vi "3DOFChairControlRebuild.vi"(9 "Scaling Factor":i32=10, 10 "Current Coord":cluster{"x (mm)":dbl, "y (mm)":dbl}={"x (mm)"=-200.0, "y (mm)"=200.0}, 11 "Previous Coord":cluster{"x (mm)":dbl, "y (mm)":dbl}) -> (0 "2D Picture 2":picture, 1 "theta3":dbl=nan, 2 "theta2":dbl=nan, 3 "theta1":dbl=nan)   [LabVIEW 2024]
uses:
  <userlib>/SerialVIs/subs/portX.xctl
panel:
  out "Coords for Sim":dbl[][](array[numeric])=[[-83.72269481496227, 7.427522229338194], [-60.199998575251854, 103.32411915468035], [-140.03201198405128, 16.093208020279867], [-16.82765846644173, 5.829527542811121], [34.47637796621948, -131.42242211582163], [68.40773502811334, 59.4509273398248], [141.31983353358055, 21.39471366409613], [101.5494686808696, 72.90895747770806], [-106.74616173728506, 110.28365634864979], [-65.90786459398325, 103.0414116639924], [-153.25841815303286, 18.106369867448336], [-11.71245505129427, 112.39652890839193], [20.969703171021592, 37.88273640369408]]
  out "output cluster":cluster{"x (mm)":dbl, "y (mm)":dbl}={"x (mm)"=-118.0, "y (mm)"=118.0}
  out "Array":dbl[](array[numeric])=[-118.0, 118.0]
  in  "Chair Back L":dbl=40.0
  out "result string 2":string="servo1.write(NaN)\nservo2.write(NaN)\nservo3.write(NaN)"
  in  "Chair Seat L":dbl=40.0
  in  "L 1":dbl=80.0
  in  "L2":dbl=80.0
  out "Interpolated Coords":dbl[][](array[numeric])=[[0.0, 0.0], [-2.0, 2.0], [-4.0, 4.0], [-6.0, 6.0], [-8.0, 8.0], [-10.0, 10.0], [-12.0, 12.0], [-14.000000000000002, 14.000000000000002], [-16.0, 16.0], [-18.0, 18.0], [-20.0, 20.0], [-22.0, 22.0], [-24.0, 24.0], [-26.0, 26.0], [-28.000000000000004, 28.000000000000004], [-30.0, 30.0], [-32.0, 32.0], [-34.0, 34.0], [-36.0, 36.0], [-38.0, 38.0], [-40.0, 40.0], [-42.0, 42.0], [-44.0, 44.0], [-46.0, 46.0], [-48.0, 48.0], [-50.0, 50.0], [-52.0, 52.0], [-54.0, 54.0], [-56.00000000000001, 56.00000000000001], [-57.99999999999999, 57.99999999999999], [-60.0, 60.0], [-62.0, 62.0], [-64.0, 64.0], [-66.0, 66.0], [-68.0, 68.0], [-70.0, 70.0], [-72.0, 72.0], [-74.0, 74.0], [-76.0, 76.0], [-78.0, 78.0], [-80.0, 80.0], [-82.0, 82.0], [-84.0, 84.0], [-86.0, 86.0], [-88.0, 88.0], [-90.0, 90.0], [-92.0, 92.0], [-94.0, 94.0], [-96.0, 96.0], [-98.0, 98.0], [-100.0, 100.0], [-102.0, 102.0], [-104.0, 104.0], [-106.0, 106.0], [-108.0, 108.0], [-110.00000000000001, 110.00000000000001], [-112.00000000000001, 112.00000000000001], [-113.99999999999999, 113.99999999999999], [-115.99999999999999, 115.99999999999999], [-118.0, 118.0], [-120.0, 120.0], [-122.0, 122.0], [-124.0, 124.0], [-126.0, 126.0], [-128.0, 128.0], [-130.0, 130.0], [-132.0, 132.0], [-134.0, 134.0], [-136.0, 136.0], [-138.0, 138.0], [-140.0, 140.0], [-142.0, 142.0], [-144.0, 144.0], [-146.0, 146.0], [-148.0, 148.0], [-150.0, 150.0], [-152.0, 152.0], [-154.0, 154.0], [-156.0, 156.0], [-158.0, 158.0], [-160.0, 160.0], [-162.0, 162.0], [-164.0, 164.0], [-166.0, 166.0], [-168.0, 168.0], [-170.0, 170.0], [-172.0, 172.0], [-174.0, 174.0], [-176.0, 176.0], [-178.0, 178.0], [-180.0, 180.0], [-182.0, 182.0], [-184.0, 184.0], [-186.0, 186.0], [-188.0, 188.0], [-190.0, 190.0], [-192.0, 192.0], [-194.0, 194.0], [-196.0, 196.0], [-198.0, 198.0], [-200.0, 200.0]]
  in  "portX":refnum<visa-resource-name>(xcontrol)="ASRL4"
  out "reply":string="\r\n>>> \r\n>>> "
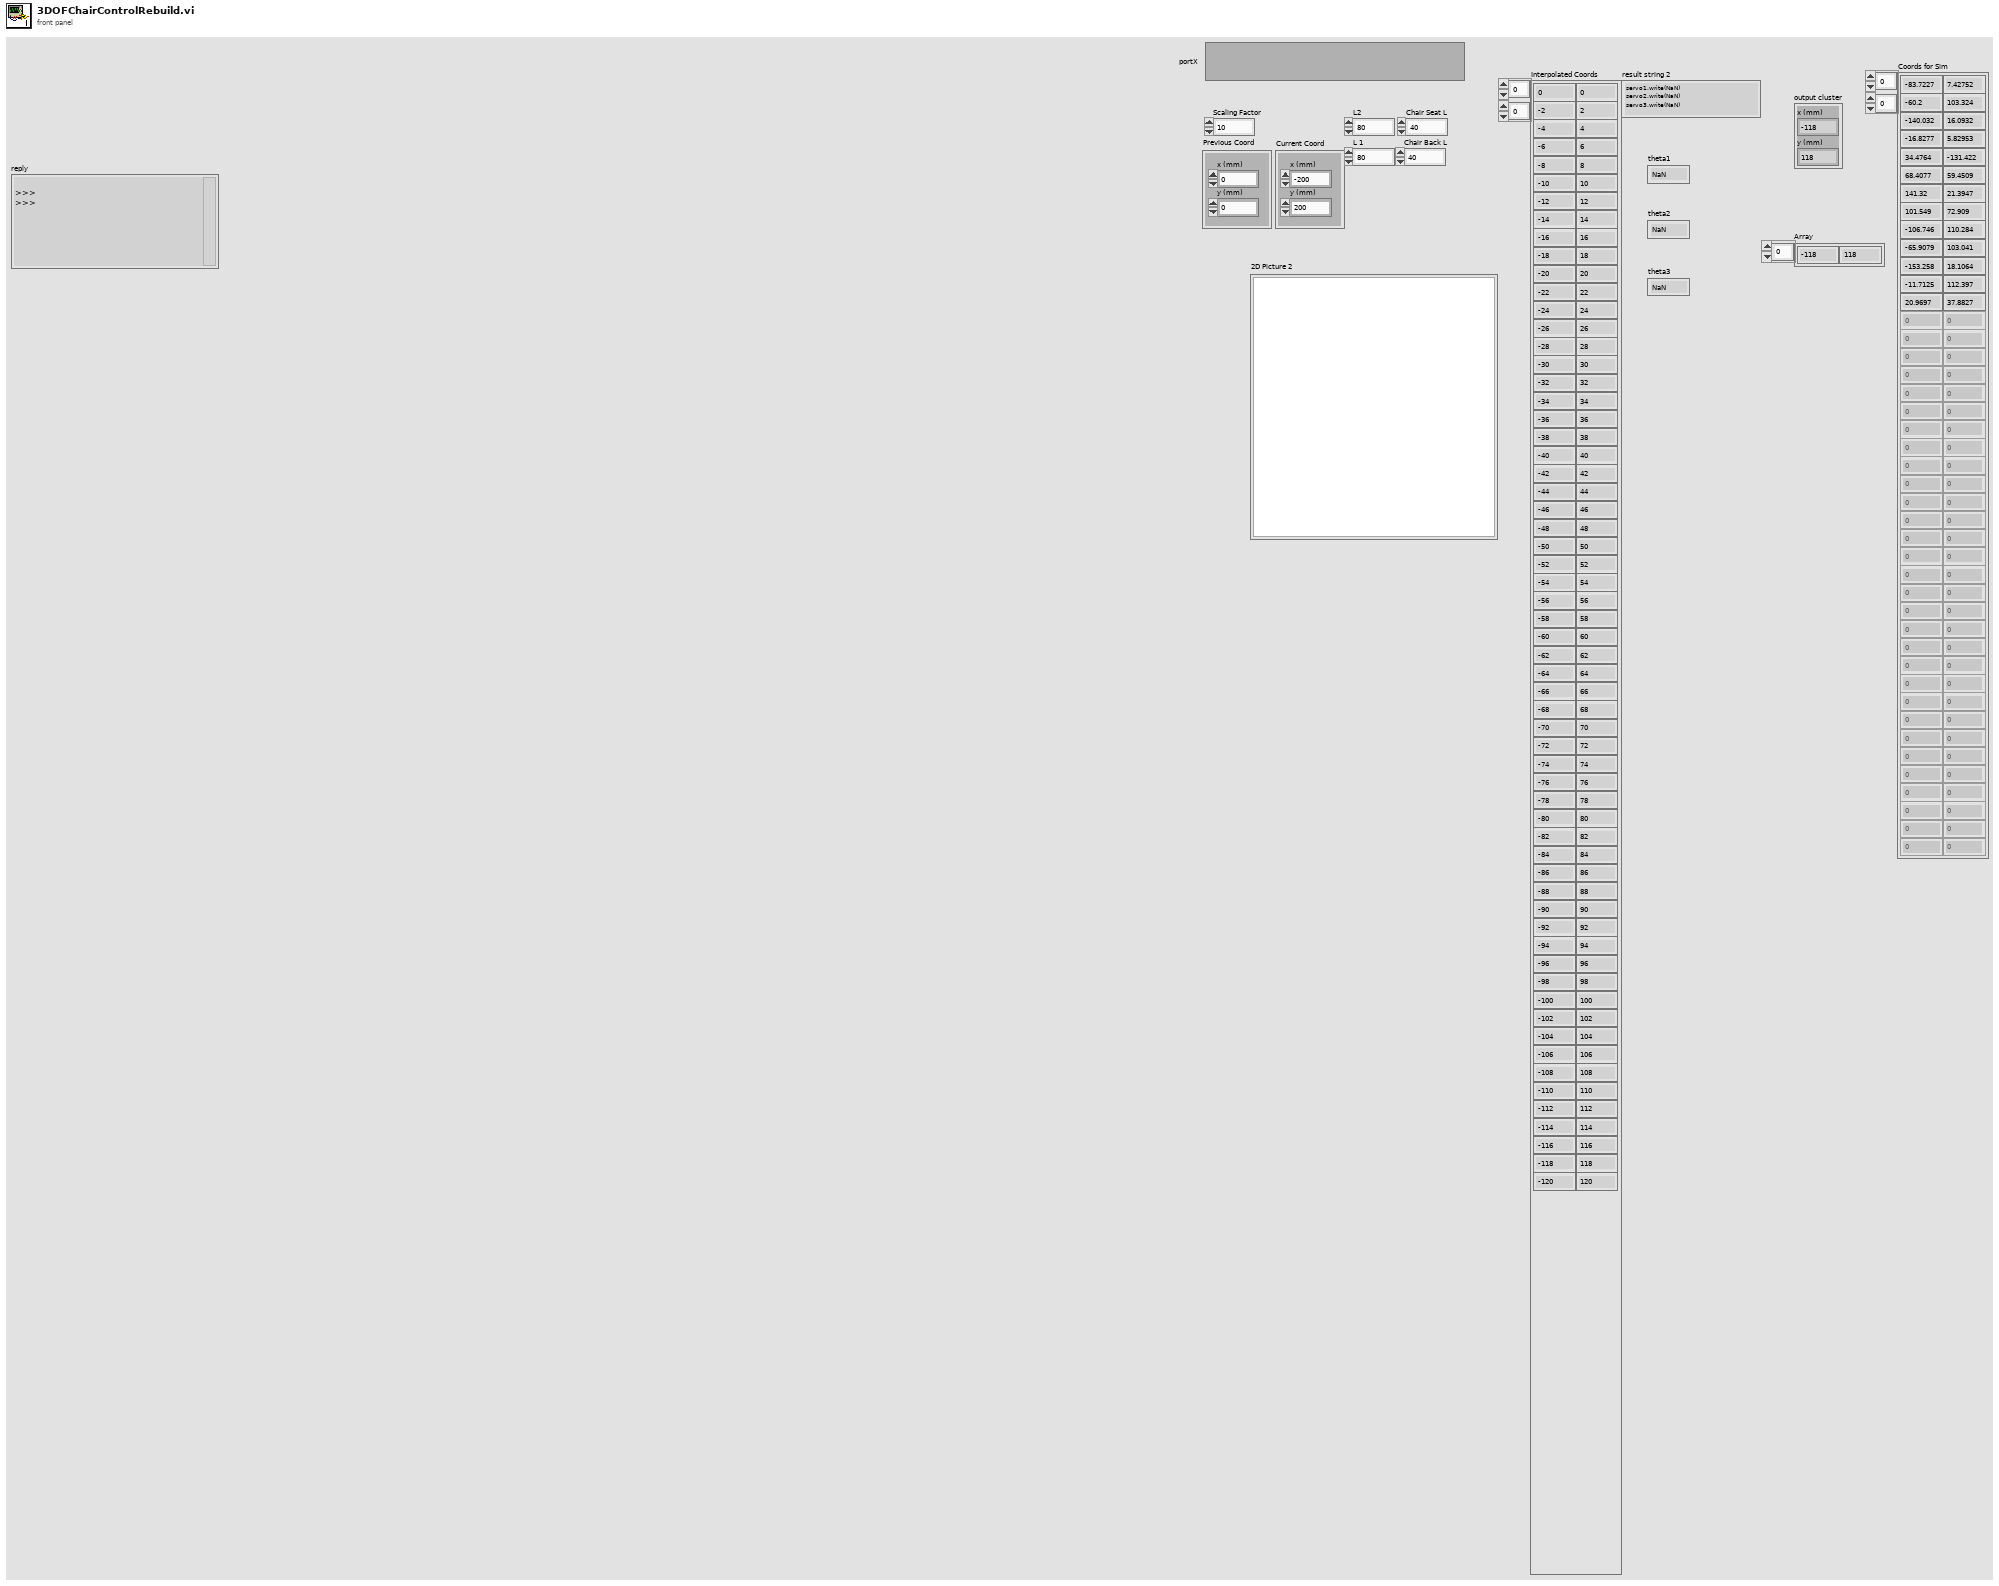
[diagram p1: front panel]
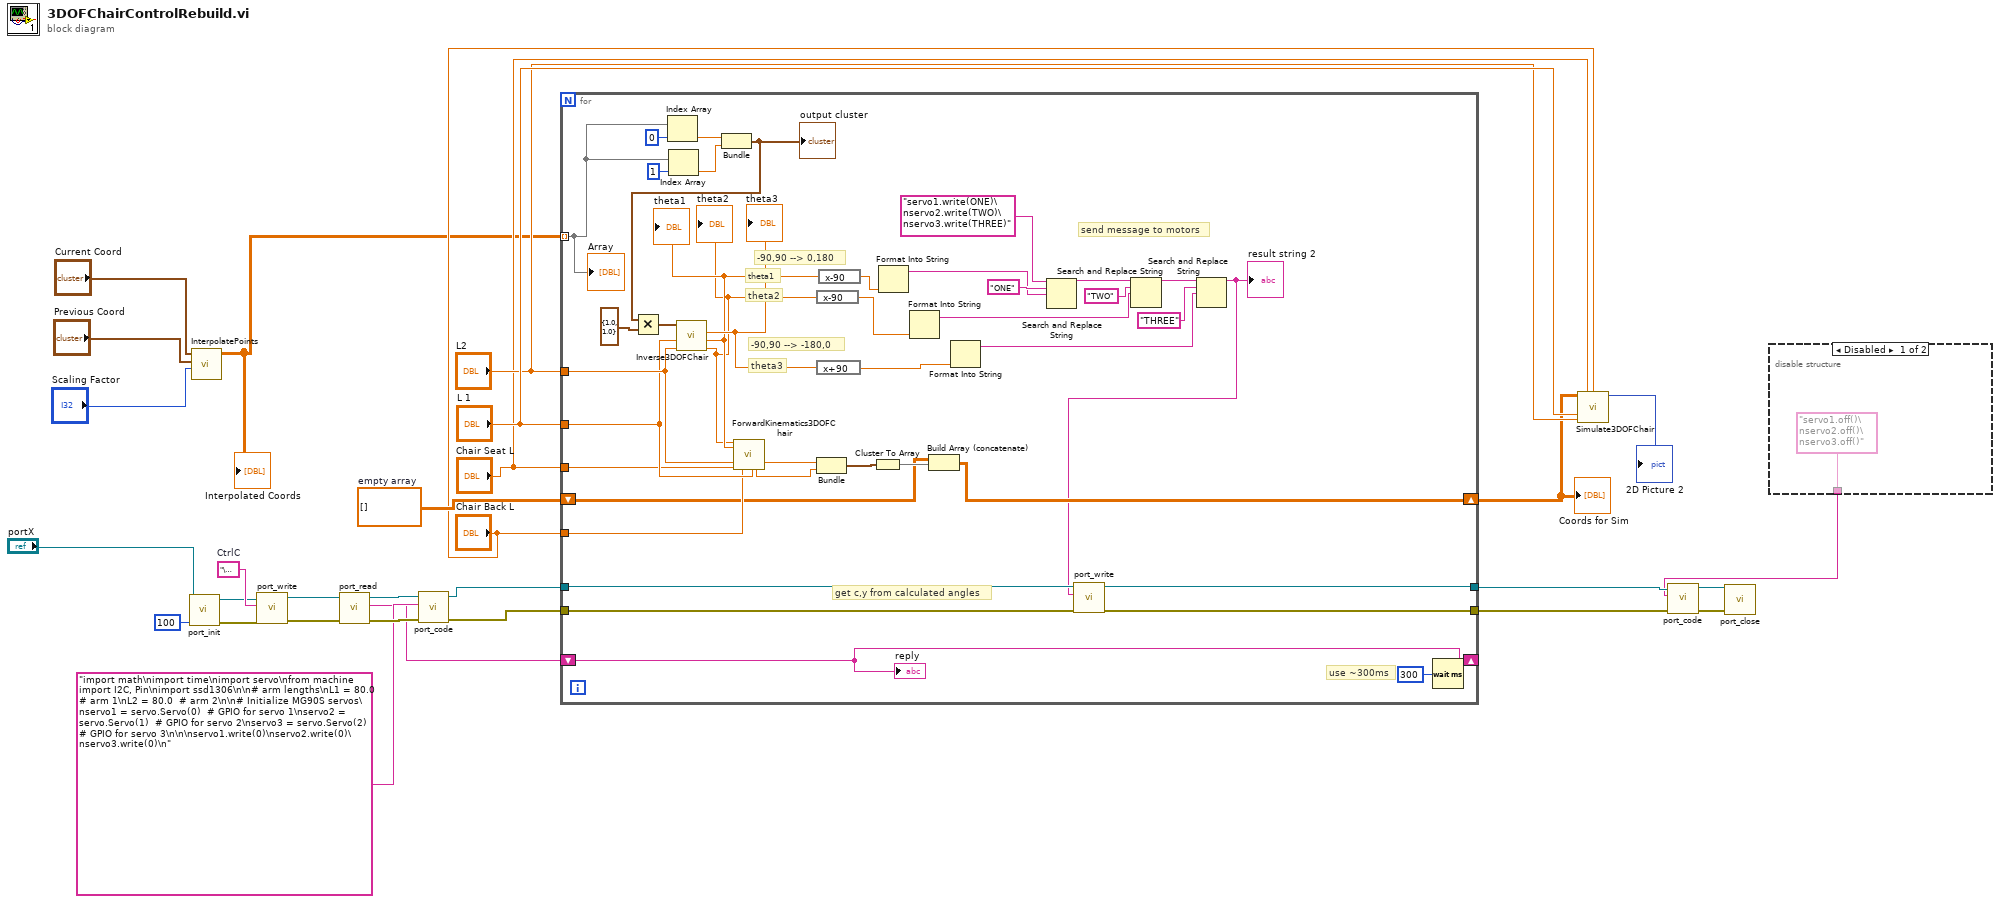
[diagram p0: block diagram]
diagram:
  w9 = dbl[][] []  # empty array
  w29 = "\u0003"  # CtrlC
  n1 = call <userlib>:"port_init.vi"("Timeout (ms)"=u32 100, "VISA Refnum in"="portX") -> ("error out"=w28:errorcluster, "VISA Refnum out"=w21:refnum<visa-resource-name>)  [unwired: 8 in]
  n2 = call "InterpolatePoints.vi"("Scaling Factor"="Scaling Factor", "Previous Coord"="Previous Coord", "Current Coord"="Current Coord") -> ("Array"=w4:dbl[][])  [unwired: 8 in]
  "Interpolated Coords" <- w4
  n3 = call <userlib>:"port_write.vi"("error in (no error)"=w28, "write buffer"=w29, "VISA Refnum in"=w21) -> ("error out"=w26:errorcluster, "VISA Refnum out"=w27:refnum<visa-resource-name>)  [unwired: 7 in]
  n4 = call <userlib>:"port_read.vi"("error in (no error)"=w26, "VISA Refnum in"=w27) -> ("error out"=w23:errorcluster, "reply"=w17:string, "VISA Refnum out"=w22:refnum<visa-resource-name>)  [unwired: 7 in]
  n5 = call <userlib>:"port_code.vi"("error in (no error)"=w23, "Code to run"="import math\nimport time\nimport servo\nfrom machine import I2C, Pin\nimport ssd1306\n\n# arm lengths\nL1 = 80.0  # arm 1\nL2 = 80.0  # arm 2\n\n# Initialize MG90S servos\nservo1 = servo.Servo(0)  # GPIO for servo 1\nservo2 = servo.Servo(1)  # GPIO for servo 2\nservo3 = servo.Servo(2)  # GPIO for servo 3\n\n\nservo1.write(0)\nservo2.write(0)\nservo3.write(0)\n", "VISA Refnum in"=w22) -> ("error out"=w18:errorcluster, "VISA Refnum out"=w19:refnum<visa-resource-name>)  [unwired: 7 in]
  n6 = for {
    tunnel: w19 -> [w67]
    tunnel: w18 -> [w66]
    tunnel: [w64] -> w14
    tunnel: [w65] -> w13
    shift-right: [w68] -> _
    shift-left: w17 -> [w68]
    tunnel: "L 1" -> [w46]
    tunnel: "L2" -> [w47]
    tunnel: "Chair Back L" -> [w45]
    tunnel: "Chair Seat L" -> [w44]
    tunnel: w4 -> [w38] mode=indexing
    shift-right: [w34] -> w3
    shift-left: w9 -> [w41]
    # "send message to motors"
    # "-90,90 --> 0,180"
    # "-90,90 --> -180,0"
    # "theta3"
    # "theta1"
    # "theta2"
    # "use ~300ms"
    # "get c,y from calculated angles"
    n7 = Index Array(array=w38, index=0) -> (element=w37:dbl)
    n8 = Index Array(array=w38, index=1) -> (element=w36:dbl)
    n9 = Bundle("y (mm)"=w37, "y (mm)"=w36) -> (w35:cluster{"y (mm)":dbl, "y (mm)":dbl})  [unwired: 1 in]
    "output cluster" <- w35
    n10 = Multiply(x=w35, y=cluster{dbl, dbl} {1.0, 1.0}) -> (x*y=w62:cluster{dbl, dbl})
    n11 = call "Inverse3DOFChair.vi"("L 2"=w47, "L 1"=w46, "end effector"=w62) -> ("theta2"=w31:dbl, "theta1"=w48:dbl, "theta3"=w61:dbl)  [unwired: 6 in]
    "theta1" <- w48
    "theta2" <- w31
    "theta3" <- w61
    n12 = call "ForwardKinematics3DOFChair.vi"("theta2"=w31, "theta1"=w48, "L2"=w47, "seat"=w44, "back"=w45, "L1"=w46) -> ("y2"=w32:dbl, "x2"=w33:dbl)  [unwired: 6 in, 6 out]
    n13 = expression code="x-90"(w31) -> (w50:dbl)
    n14 = expression code="x+90"(w61) -> (w49:dbl)
    n15 = Bundle("x2"=w33, "y2"=w32) -> (w43:cluster{"x2":dbl, "y2":dbl})  [unwired: 1 in]
    n16 = expression code="x-90"(w48) -> (w51:dbl)
    n17 = Cluster To Array(cluster=w43) -> (array=w42:dbl[])
    n18 = Format Into String(w51) -> (resulting string=w56:string)  [unwired: 3 in, 1 out]
    n19 = Format Into String "Format Into String"(w50) -> (resulting string=w55:string)  [unwired: 3 in, 1 out]
    n20 = Build Array (concatenate)(w41, w42) -> (w34:dbl[][])
    n21 = Format Into String "Format Into String"(w49) -> (resulting string=w52:string)  [unwired: 3 in, 1 out]
    n22 = Search and Replace String(input string="servo1.write(ONE)\nservo2.write(TWO)\nservo3.write(THREE)", search string="ONE", replace string=w56) -> (result string=w57:string)  [unwired: 5 in, 3 out]
    n23 = Search and Replace String(input string=w57, search string="TWO", replace string=w55) -> (result string=w53:string)  [unwired: 5 in, 3 out]
    n24 = Search and Replace String(input string=w53, search string="THREE", replace string=w52) -> (result string=w30:string)  [unwired: 5 in, 3 out]
    "result string 2" <- w30
    n25 = call <userlib>:"port_write.vi"("error in (no error)"=w66, "write buffer"=w30, "VISA Refnum in"=w67) -> ("error out"=w64:errorcluster, "VISA Refnum out"=w65:refnum<visa-resource-name>)  [unwired: 7 in]
    n26 = Wait (ms)(milliseconds to wait=u32 300) -> ()  [unwired: 1 out]
    "reply" <- w68
    "Array" <- w38
  }
  "Coords for Sim" <- w3
  n27 = call "Simulate3DOFChair.vi"("array"=w3, "L_seat"="Chair Seat L", "L_back"="Chair Back L", "L1"="L 1", "L2"="L2") -> ("2D Picture 2"=→"2D Picture 2":picture)  [unwired: 9 in, 1 out]
  n28 = disable-structure shown="Disabled" {
    disable-tunnel: ["servo1.off()\nservo2.off()\nservo3.off()" ("Code to run") _] -> w1
    frame Disabled {
    }
    frame Enabled {
    }
  }
  n29 = call <userlib>:"port_code.vi"("error in (no error)"=w14, "Code to run"=w1, "VISA Refnum in"=w13) -> ("error out"=w15:errorcluster, "VISA Refnum out"=w16:refnum<visa-resource-name>)  [unwired: 7 in]
  n30 = call <userlib>:"port_close.vi"("error in (no error)"=w15, "VISA Refnum in"=w16) -> ()  [unwired: 10 in]
